vi "Is VI-LIB__ogtk.vi"(8 "error in (no error)":errorcluster, 11 "VI reference":refnum<vi>) -> (0 "error out":errorcluster, 2 "is vi.lib?":bool, 3 "dup VI reference":refnum<vi>)   [LabVIEW 2014]
doc: "Checks if a VI's path is in vi.lib dir or subDir."
panel:
  # "is vi-lib.vi\n\nChecks if a VI's path is in vi.lib dir or subDir\n\nPlease visit http://www.OpenG.org to learn about the\nOpen Source LabVIEW software movement.\n\nNOTICE -- YOU MUST LEAVE THIS NOTICE IN PLACE.  PER THE TERMS OF THE LICENSE BELOW, YOU MAY SUBLICENSE THIS SOFTWARE \nIN ANY WAY THAT DOES NOT CONFLICT WITH THIS LICENSE.\n\n### BSD License (http://www.opensource.org/licenses/bsd-license.php) Begin ###\n \nCopyright (c) 2002, Jim Kring <jim@jimkring.com>\n\nAll rights reserved.\n\nRedistribution and use in source and binary forms, with or without modification, are permitted provided that the following conditions are met:\n\n    * Redistributions of source code must retain the above copyright notice, this list of conditions and the following disclaimer.\n    * Redistributions in binary form must reproduce the above copyright notice, this list of conditions and the following disclaimer in the \n       documentation and/or other materials provided with the distribution.\n    * Neither the name of SciWare, James Kring, Inc., nor the names of its contributors may be used to endorse or promote products derived \n       from this software without specific prior written permission.\n\nTHIS SOFTWARE IS PROVIDED BY THE COPYRIGHT HOLDERS AND CONTRIBUTORS \"AS IS\" AND ANY EXPRESS OR IMPLIED WARRANTIES, \nINCLUDING, BUT NOT LIMITED TO, THE IMPLIED WARRANTIES OF MERCHANTABILITY AND FITNESS FOR A PARTICULAR PURPOSE ARE \nDISCLAIMED. IN NO EVENT SHALL THE COPYRIGHT OWNER OR CONTRIBUTORS BE LIABLE FOR ANY DIRECT, INDIRECT, INCIDENTAL,\n SPECIAL, EXEMPLARY, OR CONSEQUENTIAL DAMAGES (INCLUDING, BUT NOT LIMITED TO, PROCUREMENT OF SUBSTITUTE GOODS OR \nSERVICES; LOSS OF USE, DATA, OR PROFITS; OR BUSINESS INTERRUPTION) HOWEVER CAUSED AND ON ANY THEORY OF LIABILITY, \nWHETHER IN CONTRACT, STRICT LIABILITY, OR TORT (INCLUDING NEGLIGENCE OR OTHERWISE) ARISING IN ANY WAY OUT OF THE USE \nOF THIS SOFTWARE, EVEN IF ADVISED OF THE POSSIBILITY OF SUCH DAMAGE.\n\n### BSD License End ###"
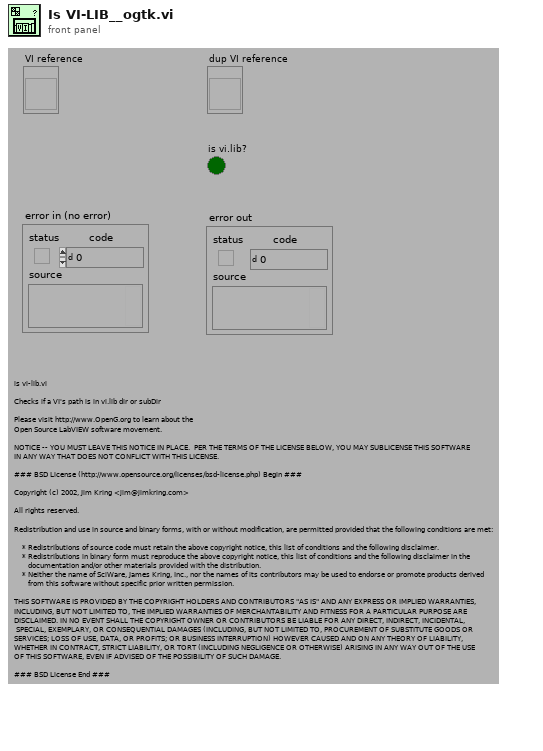
[diagram p1: front panel]
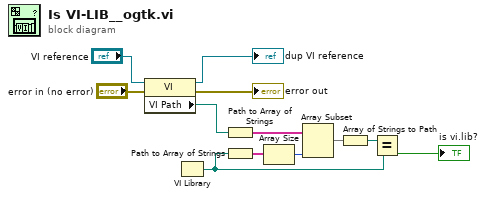
[diagram p0: block diagram]
diagram:
  n1 = property class="VI"(reference="VI reference", error in="error in (no error)") -> (reference out=→"dup VI reference":refnum<vi>, error out=→"error out":errorcluster, "VI Path"=w8:path)
  n2 = VI Library() -> (path=w2:path)
  n3 = Path to Array of Strings(0:w8) -> (2:w5:string[])  [unwired: 1 out]
  n4 = Path to Array of Strings(0:w2) -> (2:w7:string[])  [unwired: 1 out]
  n5 = Array Size(array=w7) -> (size(s)=w6:i32)
  n6 = Array Subset(array=w5, length=w6) -> (w4:string[])  [unwired: 1 in]
  n7 = Array of Strings to Path(0:w4) -> (2:w3:path)  [unwired: 1 in]
  n8 = Equal?(x=w3, y=w2) -> (x = y?=→"is vi.lib?":bool)
